vi "_ReloadDeviceInterface.vi"(0 "device name":string) -> (1 "error stack":string[](array[string]), 2 "success":bool=TRUE)   [LabVIEW 2014, in "tango.lvlib"]
uses:
  tango.lvlib
  tango_binding.so
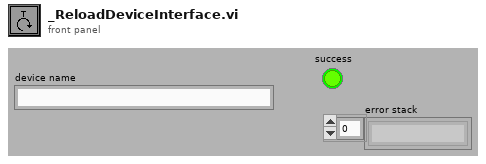
[diagram p1: front panel]
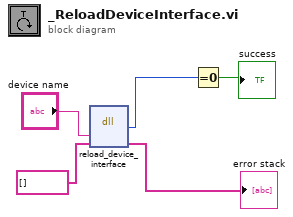
[diagram p0: block diagram]
diagram:
  n1 = dll-call lib="tango_binding.*" fn="reload_device_interface"("dev_name"="device name", "error_stack"=string[] [] ("Error Stack")) -> ("return type"=w1:i32, "error_stack"=→"error stack":string[])  [unwired: 4 in, 2 out]
  n2 = Equal To 0?(x=w1) -> (x = 0?=→"success":bool)
